vi "Correct_Fake_Origins-1.vi"(4 "error IN":errorcluster, 7 "[IN] Still connected\ntracks in group":T2) -> (0 "error OUT":errorcluster, 3 "[OUT] Clusters for Re\nconstructed Tracks":T1)   [LabVIEW 2017]
doc: "Attempt to prevent of emerging of fake origins during linking"
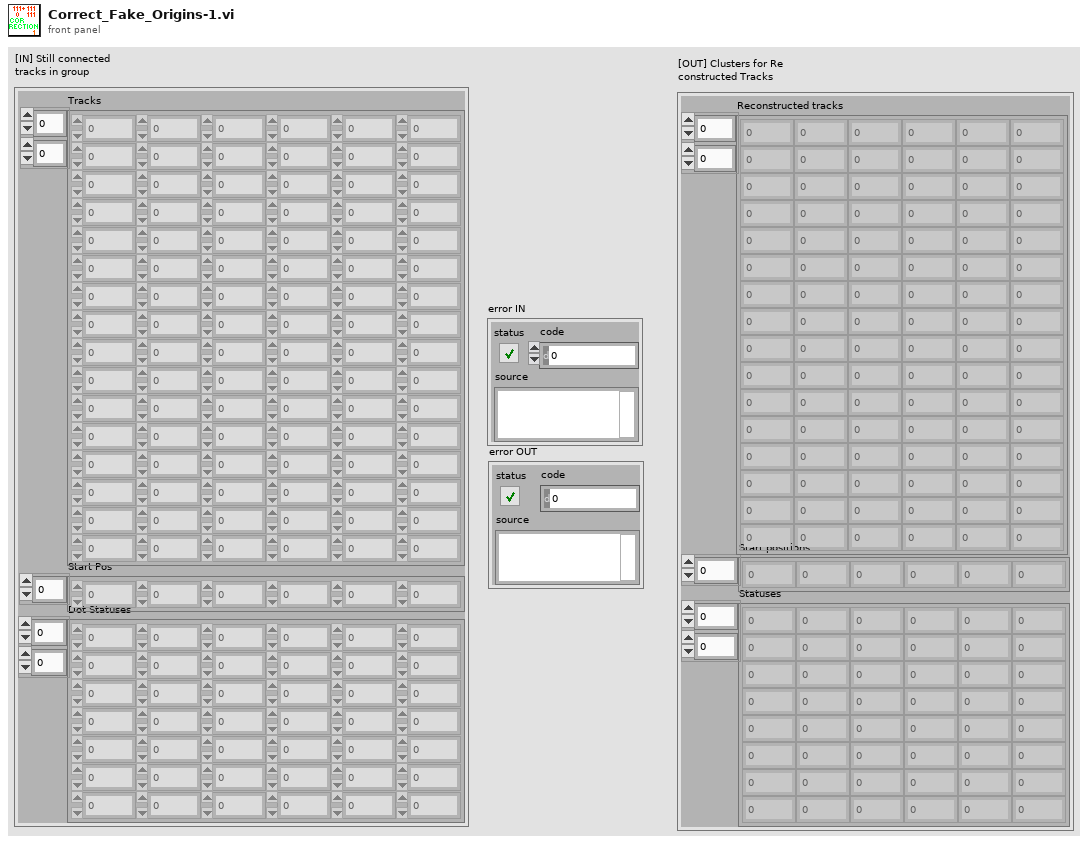
[diagram p1: front panel]
types:
  T1 = cluster{"Reconstructed tracks":dbl[][], "Start positions":i32[], "Statuses":i16[][]}
  T2 = cluster{"Tracks":dbl[][], "Start Pos":i32[], "Dot Statuses":i16[][]}
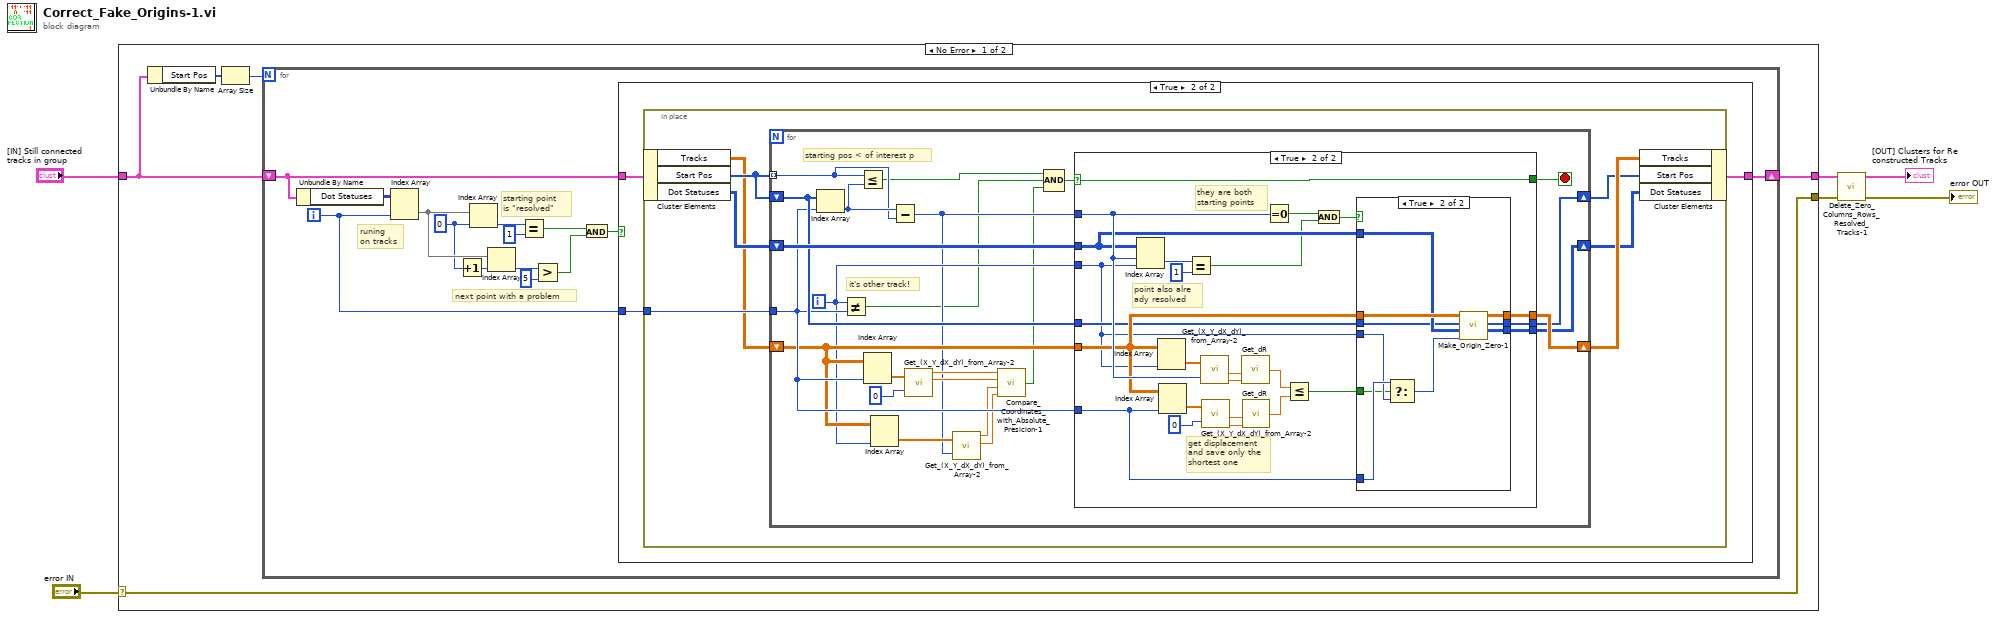
[diagram p0: block diagram]
diagram:
  n1 = case shown="No Error" "error IN" {
    selector: "error IN" -> [w8 w102]
    tunnel: "[IN] Still connected\ntracks in group" -> [w10 w103]
    tunnel: [w8 w102] -> w3
    tunnel: [w7 w103] -> w4
    frame No Error {
      n2 = Unbundle By Name(w10) -> ("Start Pos"=w11:i32[])
      n3 = Array Size(array=w11) -> (size(s)=w9:i32)
      n4 = for {
        N: w9 -> [_]
        shift-right: [w21] -> w7
        shift-left: w10 -> [w22]
        i -> [w12]
        w15 = 0
        # "starting point \nis \"resolved\""
        # "runing \non tracks"
        # "next point with a problem"
        n5 = Unbundle By Name(w22) -> ("Dot Statuses"=w23:i16[][])
        n6 = Index Array(array=w23, index (col)=w12) -> (element=w19:i16[])  [unwired: 1 in]
        n7 = Increment(x=w15) -> (x+1=w25:i32)
        n8 = Index Array(array=w19, index=w15) -> (element=w20:i16)
        n9 = Index Array(array=w19, index=w25) -> (element=w18:i16)
        n10 = Equal?(x=w20, y=i16 1) -> (x = y?=w14:bool)
        n11 = Greater?(x=w18, y=i16 5) -> (0:w13:bool)
        n12 = And(x=w14, y=w13) -> (x .and. y?=w16:bool)
        n13 = case shown="True" w16 {
          tunnel: w22 -> [w26 w29]
          tunnel: [w26 w28] -> w21
          tunnel: w12 -> [_ w27]
          frame False {
          }
          frame True {
            n14 = in-place {
              in-place-border: w27 -> [w36]
              n15 = in-place-cluster #1(w29) -> ("Tracks"=w33:dbl[][], "Start Pos"=w35:i32[], "Dot Statuses"=w34:i16[][])
              n16 = for {
                tunnel: w35 -> [w58] mode=indexing
                tunnel: w36 -> [w48]
                shift-right: [w54] -> w32
                shift-left: w33 -> [w47]
                shift-right: [w52] -> w31
                shift-left: w34 -> [w57]
                shift-right: [w53] -> w30
                shift-left: w35 -> [w56]
                i -> [w44]
                stop <- w55 stop-if-true
                # "it's other track!"
                # "starting pos < of interest p"
                n17 = Index Array(array=w56, index=w48) -> (element=w59:i32)
                n18 = Not Equal?(x=w44, y=w48) -> (x != y?=w39:bool)
                n19 = Less Or Equal?(x=w58, y=w59) -> (x <= y?=w40:bool)
                n20 = Index Array(array=w47, index (col)=w48) -> (element=w51:dbl[])  [unwired: 1 in]
                n21 = Index Array(array=w47, index (col)=w44) -> (element=w45:dbl[])  [unwired: 1 in]
                n22 = Subtract(x=w59, y=w58) -> (x-y=w43:i32)
                n23 = call "Get_(X_Y_dX_dY)_from_Array-2.vi"("(X,Y,dX,dY)"=w51, "Index of Displacement"=0) -> ("X"=w50:dbl, "Y"=w49:dbl)  [unwired: 2 out]
                n24 = call "Get_(X_Y_dX_dY)_from_Array-2.vi"("(X,Y,dX,dY)"=w45, "Index of Displacement"=w43) -> ("X"=w42:dbl, "Y"=w41:dbl)  [unwired: 2 out]
                n25 = call "Compare_Coordinates_with_Absolute_Presicion-1.vi"("X 1"=w50, "Y 1"=w49, "X 2"=w42, "Y 2"=w41) -> ("[OUT] Same coordinates?"=w37:bool)  [unwired: 1 in]
                n26 = Compound Arithmetic op=AND(w40, w39, w37) -> (w38:bool)
                n27 = case shown="True" w38 {
                  selector: w38 -> [w61 w71]
                  tunnel: w43 -> [_ w77]
                  tunnel: w57 -> [w60 w75]
                  tunnel: w44 -> [_ w72]
                  tunnel: w47 -> [w63 w76]
                  tunnel: w48 -> [_ w74]
                  tunnel: w56 -> [w62 w73]
                  tunnel: [w61 w71] -> w55
                  tunnel: [w63 w70] -> w54
                  tunnel: [w62 w69] -> w53
                  tunnel: [w60 w68] -> w52
                  frame False {
                  }
                  frame True {
                    # "they are both \nstarting points"
                    # "get displacement\nand save only the\nshortest one"
                    # "point also alre\nady resolved"
                    n28 = Index Array(array=w75, index (row)=w77, index (col)=w72) -> (element=w87:i16)
                    n29 = Index Array(array=w76, index (col)=w72) -> (element=w86:dbl[])  [unwired: 1 in]
                    n30 = Index Array(array=w76, index (col)=w74) -> (element=w83:dbl[])  [unwired: 1 in]
                    n31 = Equal?(x=w87, y=i16 1) -> (x = y?=w66:bool)
                    n32 = call "Get_(X_Y_dX_dY)_from_Array-2.vi"("(X,Y,dX,dY)"=w86, "Index of Displacement"=w77) -> ("dX"=w85:dbl, "dY"=w84:dbl)  [unwired: 2 out]
                    n33 = call "Get_(X_Y_dX_dY)_from_Array-2.vi"("(X,Y,dX,dY)"=w83, "Index of Displacement"=0) -> ("dX"=w81:dbl, "dY"=w80:dbl)  [unwired: 2 out]
                    n34 = call "Get_dR.vi"("[IN] dY"=w84, "[IN] dX"=w85) -> ("[OUT] dR"=w79:dbl)  [unwired: 2 in]
                    n35 = call "Get_dR.vi"("[IN] dY"=w80, "[IN] dX"=w81) -> ("[OUT] dR"=w78:dbl)  [unwired: 2 in]
                    n36 = Equal To 0?(x=w77) -> (x = 0?=w67:bool)
                    n37 = Less Or Equal?(x=w79, y=w78) -> (x <= y?=w65:bool)
                    n38 = And(x=w67, y=w66) -> (x .and. y?=w64:bool)
                    n39 = case shown="True" w64 {
                      tunnel: w76 -> [w91 w101]
                      tunnel: w75 -> [w89 w100]
                      tunnel: w74 -> [_ w98]
                      tunnel: w73 -> [w90 w99]
                      tunnel: w72 -> [_ w97]
                      tunnel: [w91 w95] -> w70
                      tunnel: [w90 w94] -> w69
                      tunnel: [w89 w93] -> w68
                      tunnel: w65 -> [_ w92]
                      frame False {
                      }
                      frame True {
                        n40 = Select(t=w98, s=w92, f=w97) -> (s? t:f=w96:i32)
                        n41 = call "Make_Origin_Zero-1.vi"("[IN] # Track"=w96, "[IN] Dot Statuses"=w100, "[IN] Start Pos"=w99, "[IN] Tracks"=w101) -> ("[OUT] Statuses"=w93:i16[][], "[OUT] Start Pos"=w94:i32[], "[OUT] Tracks"=w95:dbl[][])  [unwired: 1 in]
                      }
                    }
                  }
                }
              }
              n42 = in-place-cluster #1("Tracks"=w32, "Start Pos"=w30, "Dot Statuses"=w31) -> (w28:T2)
            }
          }
        }
      }
    }
    frame Error {
    }
  }
  n43 = call "Delete_Zero_Columns_Rows_Resolved_Tracks-1.vi"("error IN"=w3, "[IN] Clusters for Re\nconstructed Tracks"=w4) -> ("error OUT"=→"error OUT":errorcluster, "[OUT] Clusters for Re\nconstructed Tracks"=→"[OUT] Clusters for Re\nconstructed Tracks":T1)  [unwired: 4 in]
